vi "fpga_nestedFOR_W&R_ADC_W_2DACs_Write_then_CLK.vi"() -> ()   [LabVIEW 2018]
uses:
  <vilib>/rvi/Emulation/niFpgaGetClockAttributes.vi
  <vilib>/rvi/Emulation/niFpgaSctlEmulationGetInTimedLoop.vi
  <vilib>/rvi/Emulation/niFpgaEmulationReportErrorSimple.vi
  <vilib>/rvi/Emulation/niFpgaProcessEmulError.vi
  <vilib>/rvi/eio/common/nirviEmuTemplateMethod_errors.vi
  <vilib>/rvi/Emulation/niFpgaCriticalErrorInLSC.vi
  <vilib>/eio/EIONode/EIONode.xnode
panel:
  out "ADC  1 R":bool[](array[boolean])
  in  "ADC 2 W":bool[](array[boolean])=[FALSE, FALSE, FALSE, TRUE, FALSE, FALSE, FALSE, FALSE, FALSE, FALSE, FALSE, FALSE, FALSE, FALSE, FALSE, FALSE]
  in  "delay cs (uSec)":u32=20
  in  "ADC 1 W":bool[](array[boolean])=[FALSE, FALSE, FALSE, FALSE, FALSE, TRUE, FALSE, FALSE, FALSE, FALSE, FALSE, FALSE, FALSE, FALSE, FALSE, FALSE]
  in  "ADC 4 W":bool[](array[boolean])=[FALSE, FALSE, TRUE, TRUE, FALSE, FALSE, FALSE, FALSE, FALSE, FALSE, FALSE, FALSE, FALSE, FALSE, FALSE, FALSE]
  in  "ADC 3 W":bool[](array[boolean])=[FALSE, FALSE, TRUE, FALSE, FALSE, FALSE, FALSE, FALSE, FALSE, FALSE, FALSE, FALSE, FALSE, FALSE, FALSE, FALSE]
  out "i":i32=2
  out "ADC 2 R":bool[](array[boolean])
  out "ADC 4 R":bool[](array[boolean])
  out "ADC 3 R":bool[](array[boolean])
  in  "Stop":bool
  in  "DAC 1 write":bool[](array[boolean])=[TRUE, FALSE, FALSE, FALSE, FALSE, FALSE, FALSE, FALSE, FALSE, FALSE, FALSE, FALSE, FALSE, FALSE, FALSE, FALSE]
  in  "DAC 2 write":bool[](array[boolean])=[TRUE, FALSE, FALSE, FALSE, FALSE, FALSE, FALSE, FALSE, FALSE, FALSE, FALSE, FALSE, FALSE, FALSE, FALSE, FALSE]
  # "+/- 10 V"
  # "+/- 5 V"
  # "+/- 5 V"
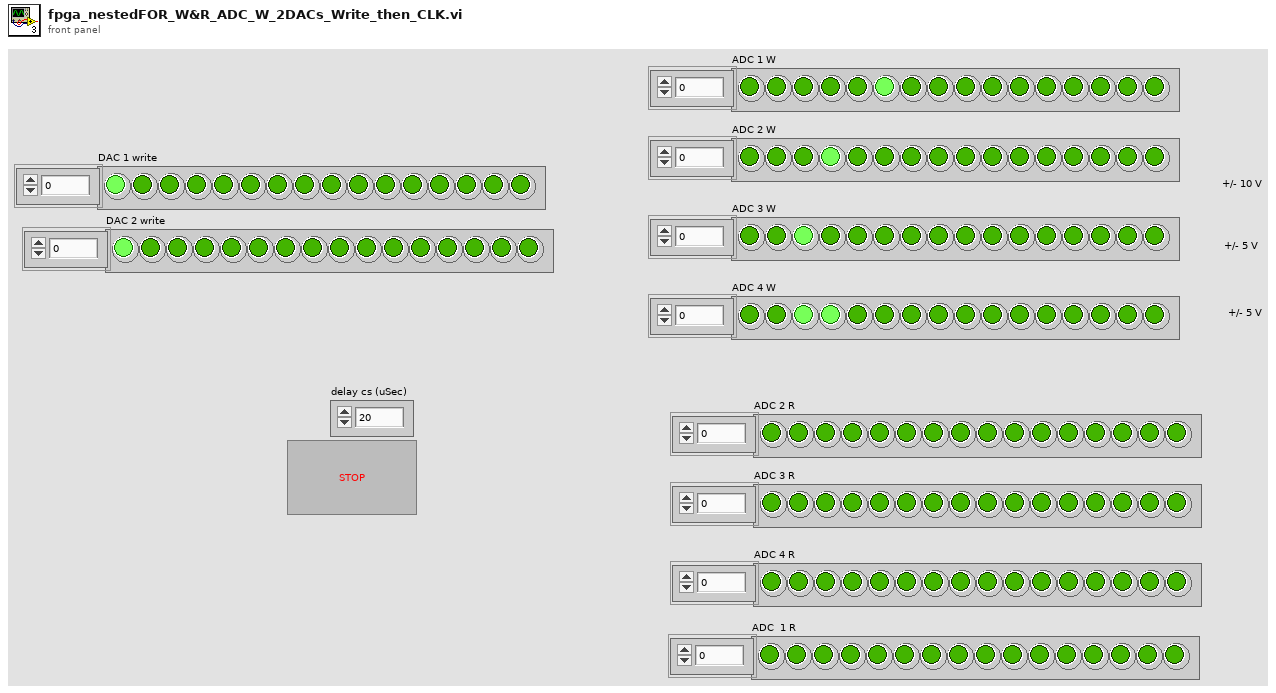
[diagram p1: front panel]
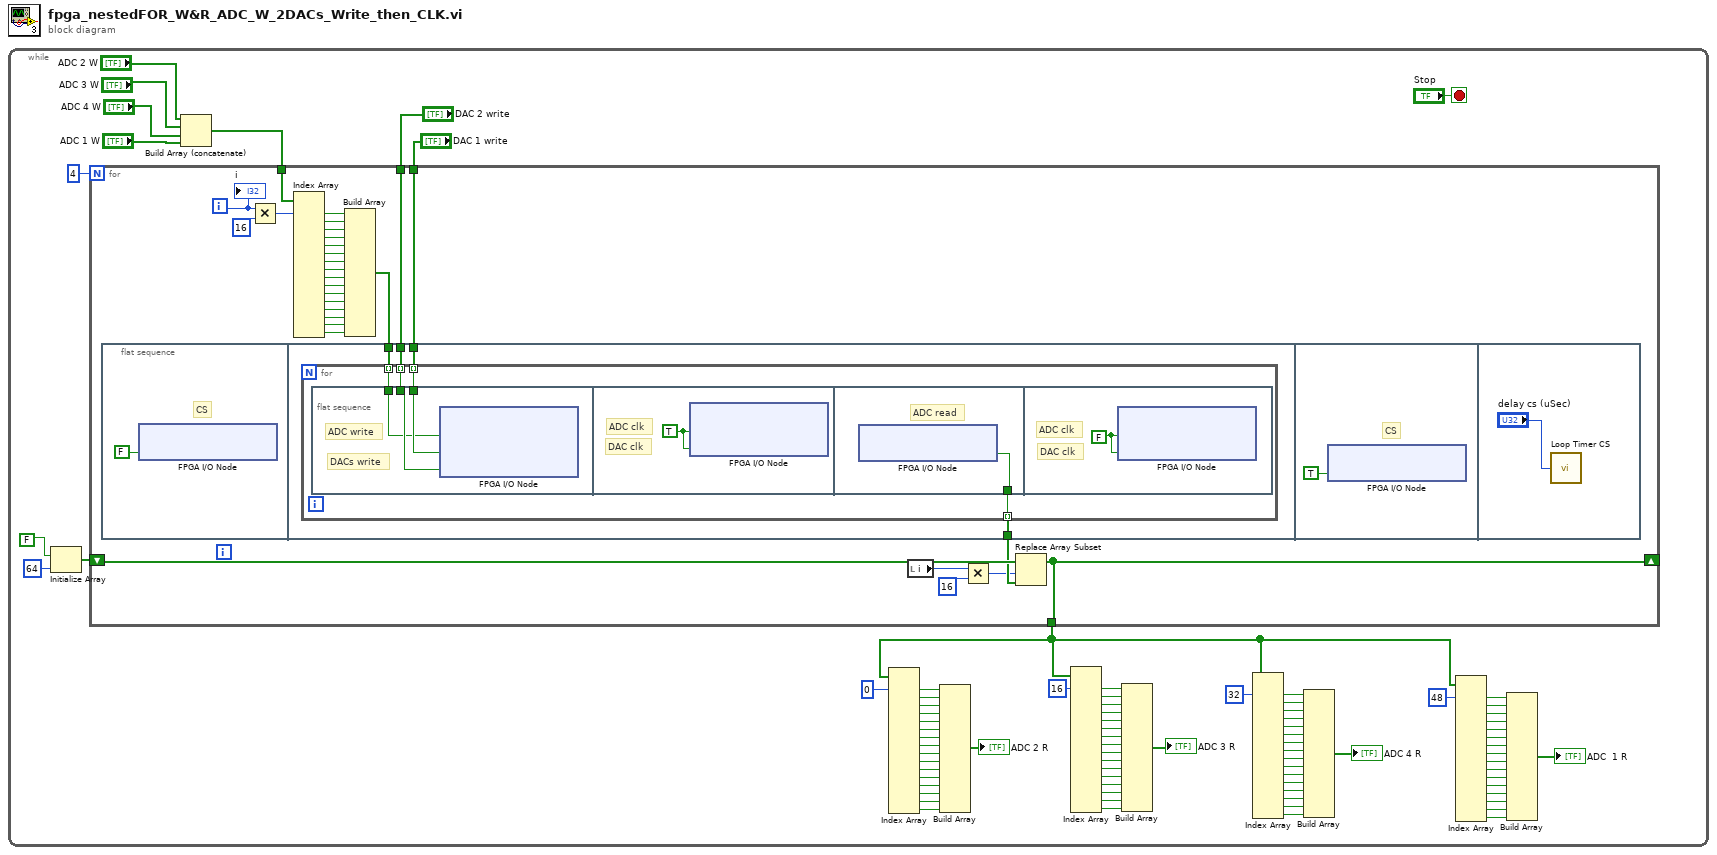
[diagram p0: block diagram]
diagram:
  n1 = while {
    stop <- "Stop" stop-if-true
    n2 = Initialize Array(FALSE, 64 ("dimension size")) -> (w65:bool[])
    n3 = Build Array (concatenate)("ADC 2 W", "ADC 3 W", "ADC 4 W", "ADC 1 W") -> (w82:bool[])
    n4 = for {
      N: 4 -> [_]
      tunnel: "DAC 2 write" -> [w114]
      tunnel: "DAC 1 write" -> [w113]
      tunnel: w82 -> [w111]
      shift-right: [w87] -> _
      shift-left: w65 -> [w92]
      tunnel: [w87] -> w1
      i -> [w86]
      n5 = flat-sequence {
        tunnel: w113 -> [w119]
        tunnel: w114 -> [w118]
        tunnel: w93 -> [w117]
        tunnel: [w116] -> w91
        frame #0 {
          # "CS"
          n6 = xnode "FPGA I/O Node"("ConnectorA/DIO4"=FALSE) -> ()  [unwired: 1 in, 1 out]
        }
        frame #1 {
          n7 = for {
            tunnel: w119 -> [w123] mode=indexing
            tunnel: w118 -> [w122] mode=indexing
            tunnel: w117 -> [w121] mode=indexing
            tunnel: [w120] -> w116 mode=indexing
            n8 = flat-sequence {
              tunnel: w123 -> [w126]
              tunnel: w122 -> [w125]
              tunnel: w121 -> [w124]
              tunnel: [w128] -> w120
              frame #0 {
                # "DACs write"
                # "ADC write"
                n9 = xnode "FPGA I/O Node"("ConnectorA/DIO2"=w124, "ConnectorA/DIO6"=w126, "ConnectorA/DIO7"=w125) -> ()  [unwired: 3 in, 3 out]
              }
              frame #1 {
                w127 = TRUE ("ConnectorA/DIO3")
                # "DAC clk"
                # "ADC clk"
                n10 = xnode "FPGA I/O Node"("ConnectorA/DIO3"=w127, "ConnectorA/DIO5"=w127) -> ()  [unwired: 2 in, 2 out]
              }
              frame #2 {
                # "ADC read"
                n11 = xnode "FPGA I/O Node"() -> ("ConnectorA/DIO1"=w128:bool)  [unwired: 1 in, 1 out]
              }
              frame #3 {
                w129 = FALSE ("ConnectorA/DIO3")
                # "DAC clk"
                # "ADC clk"
                n12 = xnode "FPGA I/O Node"("ConnectorA/DIO3"=w129, "ConnectorA/DIO5"=w129) -> ()  [unwired: 2 in, 2 out]
              }
            }
          }
        }
        frame #2 {
          # "CS"
          n13 = xnode "FPGA I/O Node"("ConnectorA/DIO4"=TRUE) -> ()  [unwired: 1 in, 1 out]
        }
        frame #3 {
          n14 = call "Loop Timer CS"("Count(uSec)"="delay cs (uSec)") -> ()  [unwired: 1 out]
        }
      }
      n15 = Multiply(x=w86, y=16) -> (x*y=w110:i32)
      n16 = Index Array(array=w111, index #1=w110) -> (element #1=w109:bool, element #2=w108:bool, element #3=w107:bool, element #4=w106:bool, element #5=w105:bool, element #6=w104:bool, element #7=w103:bool, element #8=w102:bool, element #9=w101:bool, element #10=w100:bool, element #11=w99:bool, element #12=w98:bool, element #13=w97:bool, element #14=w96:bool, element #15=w95:bool, element #16=w94:bool)  [unwired: 15 in]
      n17 = Build Array(w109, w108, w107, w106, w105, w104, w103, w102, w101, w100, w99, w98, w97, w96, w95, w94) -> (w93:bool[])
      n18 = local read "i"() -> (w89:i32)
      n19 = Multiply(x=w89, y=16) -> (x*y=w88:i32)
      n20 = Replace Array Subset(array=w92, new element=w91, index=w88) -> (w87:bool[])
      "i" <- w86
    }
    n21 = Index Array(array=w1, index #1=0 ("index")) -> (element #1=w24:bool, element #2=w25:bool, element #3=w80:bool, element #4=w79:bool, element #5=w78:bool, element #6=w77:bool, element #7=w76:bool, element #8=w75:bool, element #9=w74:bool, element #10=w73:bool, element #11=w72:bool, element #12=w71:bool, element #13=w70:bool, element #14=w69:bool, element #15=w64:bool, element #16=w63:bool)  [unwired: 15 in]
    n22 = Build Array(w24, w25, w80, w79, w78, w77, w76, w75, w74, w73, w72, w71, w70, w69, w64, w63) -> (→"ADC 2 R":bool[])
    n23 = Index Array(array=w1, index #1=16 ("index")) -> (element #1=w26:bool, element #2=w61:bool, element #3=w60:bool, element #4=w59:bool, element #5=w58:bool, element #6=w57:bool, element #7=w56:bool, element #8=w55:bool, element #9=w54:bool, element #10=w53:bool, element #11=w52:bool, element #12=w51:bool, element #13=w50:bool, element #14=w49:bool, element #15=w47:bool, element #16=w46:bool)  [unwired: 15 in]
    n24 = Build Array(w26, w61, w60, w59, w58, w57, w56, w55, w54, w53, w52, w51, w50, w49, w47, w46) -> (→"ADC 3 R":bool[])
    n25 = Index Array(array=w1, index #1=32 ("index")) -> (element #1=w27:bool, element #2=w45:bool, element #3=w44:bool, element #4=w43:bool, element #5=w42:bool, element #6=w41:bool, element #7=w40:bool, element #8=w39:bool, element #9=w38:bool, element #10=w37:bool, element #11=w36:bool, element #12=w35:bool, element #13=w34:bool, element #14=w33:bool, element #15=w31:bool, element #16=w30:bool)  [unwired: 15 in]
    n26 = Build Array(w27, w45, w44, w43, w42, w41, w40, w39, w38, w37, w36, w35, w34, w33, w31, w30) -> (→"ADC 4 R":bool[])
    n27 = Index Array(array=w1, index #1=48 ("index")) -> (element #1=w2:bool, element #2=w19:bool, element #3=w18:bool, element #4=w17:bool, element #5=w16:bool, element #6=w15:bool, element #7=w14:bool, element #8=w13:bool, element #9=w12:bool, element #10=w11:bool, element #11=w10:bool, element #12=w9:bool, element #13=w8:bool, element #14=w7:bool, element #15=w5:bool, element #16=w4:bool)  [unwired: 15 in]
    n28 = Build Array(w2, w19, w18, w17, w16, w15, w14, w13, w12, w11, w10, w9, w8, w7, w5, w4) -> (→"ADC  1 R":bool[])
  }
